vi "svc_Complex to Mag Spectrum.vi"(4 "complex spectrum":cluster{"f0":dbl, "df":dbl, "spectrum":cdb[]} {"spectrum" format="%.2f"; "df" format="%.2f"; "f0" format="%.2f"}) -> (1 "magnitude spectrum":cluster{"f0":dbl, "df":dbl, "spectrum":dbl[]} {"spectrum" format="%.2f"; "df" format="%.2f"; "f0" format="%.2f"})   [LabVIEW 2017]
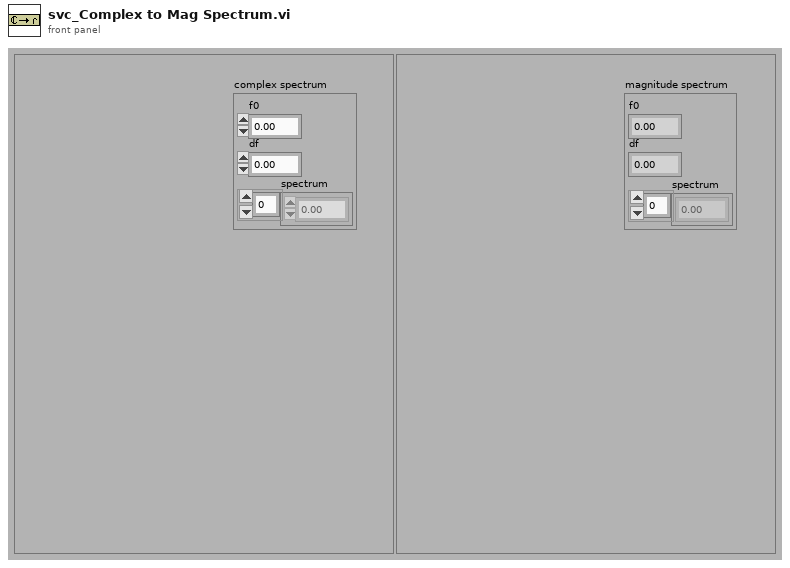
[diagram p1: front panel]
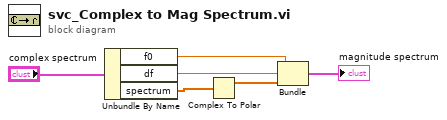
[diagram p0: block diagram]
diagram:
  n1 = Unbundle By Name("complex spectrum") -> ("f0"=w3:dbl, "df"=w4:dbl, "spectrum"=w2:cdb[])
  n2 = Complex To Polar(r * e^(i*theta)=w2) -> (r=w1:dbl[])  [unwired: 1 out]
  n3 = Bundle("f0"=w3, "df"=w4, w1) -> (→"magnitude spectrum":cluster{"f0":dbl, "df":dbl, dbl[]})  [unwired: 1 in]
